vi "AreaOfTriangle.vi"() -> ()   [LabVIEW 2023]
panel:
  out "Block Area":dbl
  out "MatLab Area":dbl
  in  "Height":dbl
  in  "Base":dbl
  # "Area Calculator: Right Triangles\nJacob Read"
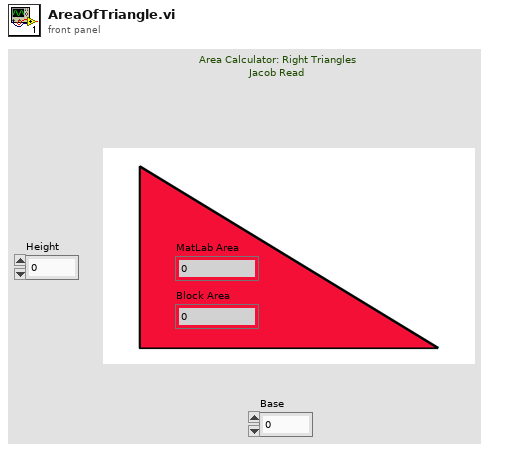
[diagram p1: front panel]
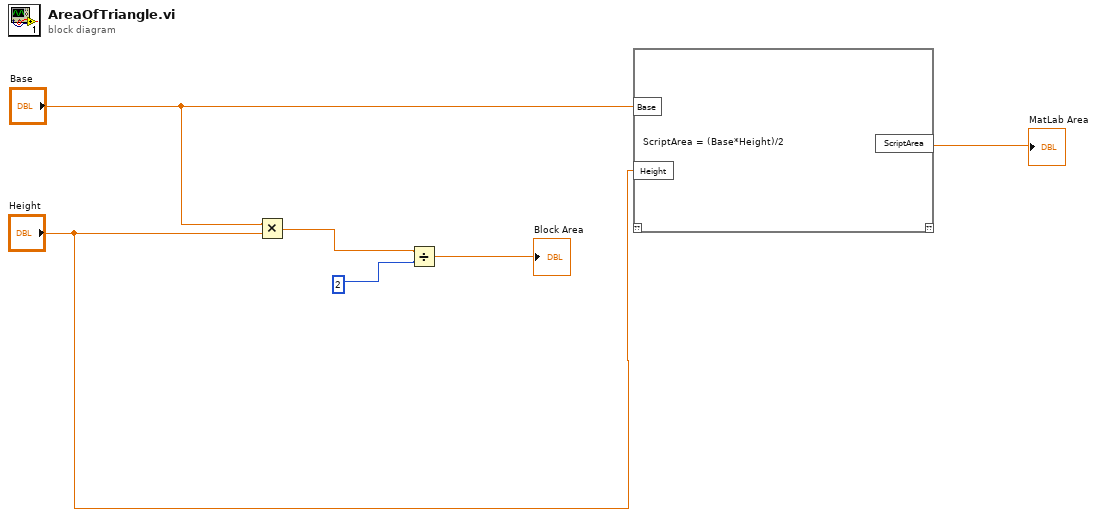
[diagram p0: block diagram]
diagram:
  n1 = Multiply(x="Base", y="Height") -> (x*y=w6:dbl)
  n2 = Divide(x=w6, y=2) -> (x/y=→"Block Area":dbl)
  n3 = script code="ScriptArea = (Base*Height)/2"("Base"="Base", "Height"="Height") -> ("ScriptArea"=→"MatLab Area":dbl)  [unwired: 1 in, 1 out]
